vi "set_config_cluster.vi"(8 "error in (no error)":errorcluster, 10 "config cluster variant":variant, 11 "ExperimentControllerDL090130Interval in":refnum<class "ExperimentControllerDL090130Interval.lvclass">) -> (0 "error out":errorcluster, 3 "ExperimentControllerDL090130Interval out":refnum<class "ExperimentControllerDL090130Interval.lvclass">)   [LabVIEW 2010, in "ExperimentControllerDL090130Interval.lvclass"]
uses:
  ExperimentControllerDL090130Interval.lvclass
  ExperimentControllerDL090130Interval.lvclass/ExperimentControllerDL090130Interval.ctl
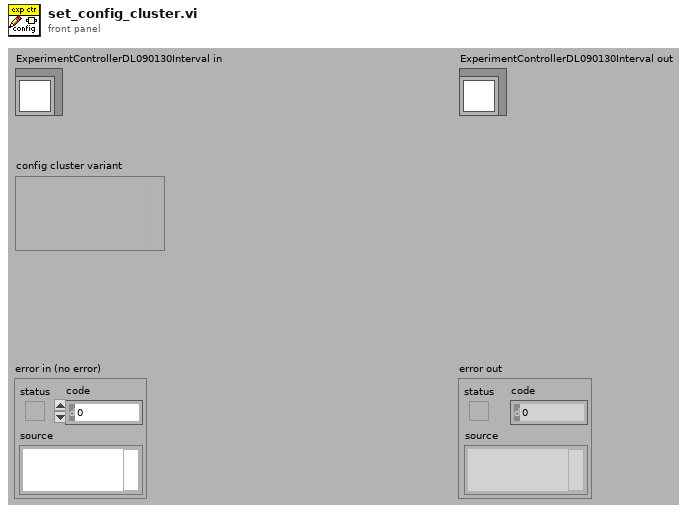
[diagram p1: front panel]
types:
  T1 = typedef "ExperimentControllerDL090130Interval.lvclass/config_data.ctl" = cluster{"sweep":T2}
  T2 = typedef "plugin_specification.ctl" = cluster{"class path":string, "configuration":string, "label":string, "settings name":string}
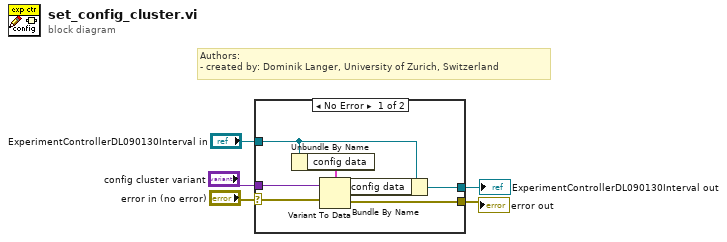
[diagram p0: block diagram]
diagram:
  # "Authors: \n- created by: Dominik Langer, University of Zurich, Switzerland"
  n1 = case shown="No Error" "error in (no error)" {
    selector: "error in (no error)" -> [w12 w13]
    tunnel: "ExperimentControllerDL090130Interval in" -> [w9 w14]
    tunnel: "config cluster variant" -> [w10 _]
    tunnel: [w7 w13] -> w2
    tunnel: [w6 w14] -> w1
    frame No Error {
      n2 = Unbundle By Name(w9) -> ("config data"=w11:T1)
      n3 = Variant To Data(error in=w12, Variant=w10, type=w11) -> (error out=w7:errorcluster, data=w8:T1)
      n4 = Bundle By Name(cluster=w9, "config data"=w8) -> (w6:refnum<class "ExperimentControllerDL090130Interval.lvclass">)
    }
    frame Error {
    }
  }
  "error out" <- w2
  "ExperimentControllerDL090130Interval out" <- w1
